vi "GEA2MessageFormatter.vi"(0 "Prefix(Send/Recv)":string, 7 "GEA2 Data In":T1 {"Command" format="%02x"; "Destination" format="%02x"; "Source" format="%02x"}, 11 "Error In":errorcluster) -> (4 "Output String":string, 15 "Error Out":errorcluster)   [LabVIEW 2016, in "GEA2_Toolkit.lvlib"]
uses:
  library/GEA2_Toolkit.lvlib
  type defs/Data In.ctl
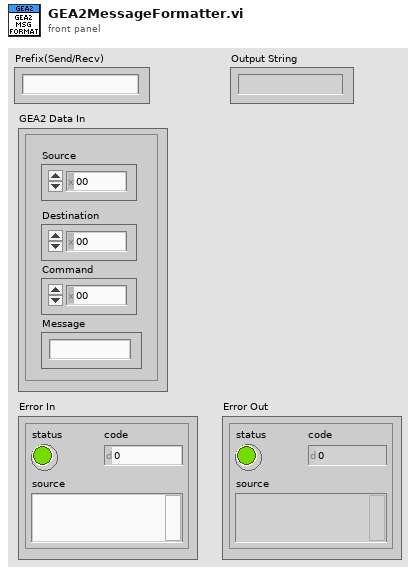
[diagram p1: front panel]
types:
  T1 = typedef "GEA2_Toolkit.lvlib/Data In.ctl" = cluster{"Source":u8, "Destination":u8, "Command":u8, "Message":string}
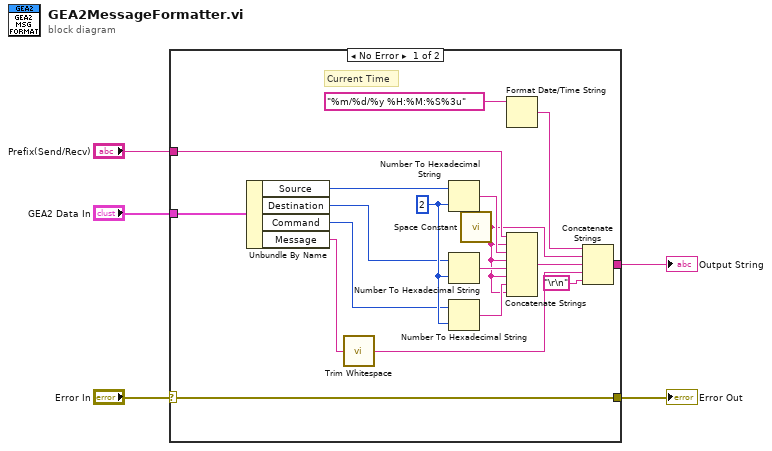
[diagram p0: block diagram]
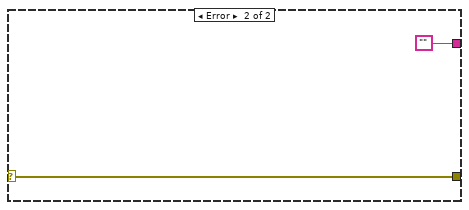
[diagram p2: hidden frame]
diagram:
  n1 = case shown="No Error" "Error In" {
    selector: "Error In" -> [w6 w25]
    tunnel: [w20 ""] -> w5
    tunnel: "Prefix(Send/Recv)" -> [w18 _]
    tunnel: "GEA2 Data In" -> [w13 _]
    tunnel: [w6 w25] -> w1
    frame No Error {
      w19 = i16 2 ("width (-)")
      # "Current Time"
      n2 = Unbundle By Name(w13) -> ("Source"=w12:u8, "Destination"=w11:u8, "Command"=w10:u8, "Message"=w8:string)
      n3 = call <vilib>:"Trim Whitespace.vi"("string"=w8) -> ("trimmed string"=w7:string)  [unwired: 1 in]
      n4 = Number To Hexadecimal String(1:w19, 2:w12) -> (0:w15:string)
      n5 = Number To Hexadecimal String(1:w19, 2:w11) -> (0:w14:string)
      n6 = Number To Hexadecimal String(1:w19, 2:w10) -> (0:w16:string)
      n7 = call <vilib>:"Space Constant.vi"() -> ("String"=w9:string)
      n8 = Format Date/Time String(time format string (%c)="%m/%d/%y %H:%M:%S%3u") -> (date/time string=w21:string)  [unwired: 2 in]
      n9 = Concatenate Strings(w18, w9, w15, w9, w14, w9, w16, w9) -> (w17:string)
      n10 = Concatenate Strings(w21, w9, w17, w7, "\r\n") -> (w20:string)
    }
    frame Error {
    }
  }
  "Output String" <- w5
  "Error Out" <- w1
